vi "Log.vi"(8 "error in (no error)":errorcluster, 10 "MB session in":refnum<class "MB_Master.lvclass">, 11 "DAM0404D in":refnum<class "DAM0404D.lvclass">) -> (0 "error out":errorcluster, 3 "DAM0404D out":refnum<class "DAM0404D.lvclass">)   [LabVIEW 2016, in "DAM0404D.lvlib" / "DAM0404D.lvclass"]
uses:
  DAM0404D.lvclass
  <vilib>/Plasmionique/MB Master/MB_Master/MB_Master.lvclass
  DAM0404D.lvclass/DAM0404D.ctl
  <vilib>/Plasmionique/MB Master/MB_ADU/MB_ADU.lvclass/MB_ADU.ctl
  <vilib>/Plasmionique/MB Master/MB_ADU/Read TX Timestamp.vi
  <vilib>/Plasmionique/MB Master/MB_ADU/Read TX Data.vi
  <vilib>/Plasmionique/MB Master/MB_ADU/Read RX Timestamp.vi
  <vilib>/Plasmionique/MB Master/MB_ADU/Read RX Data.vi
  <vilib>/Plasmionique/MB Master/MB_ADU/MB_ADU.lvclass
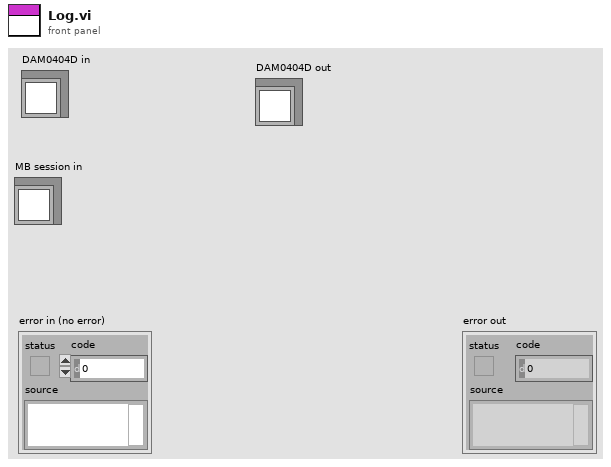
[diagram p1: front panel]
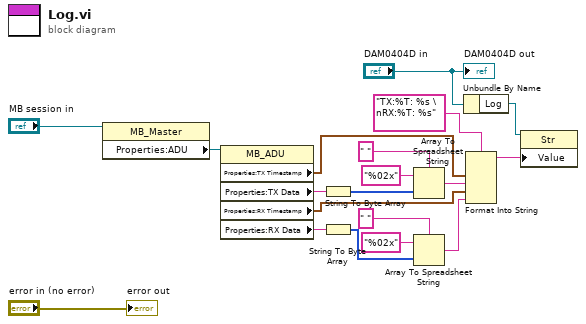
[diagram p0: block diagram]
diagram:
  n1 = property class="MB_Master"(reference="MB session in") -> ("Properties:ADU"=w18:refnum<class "MB_ADU.lvclass">)  [unwired: 1 in, 2 out]
  n2 = property class="MB_ADU"(reference=w18) -> ("Properties:TX Timestamp"=w17:timestamp, "Properties:TX Data"=w2:string, "Properties:RX Timestamp"=w16:timestamp, "Properties:RX Data"=w10:string)  [unwired: 1 in, 2 out]
  n3 = String To Byte Array(string=w2) -> (unsigned byte array=w3:u8[])
  n4 = String To Byte Array(string=w10) -> (unsigned byte array=w9:u8[])
  n5 = Array To Spreadsheet String(delimiter (Tab)=" ", array=w3, 3:"%02x" ("format string")) -> (spreadsheet string=w1:string)
  n6 = Array To Spreadsheet String(delimiter (Tab)=" ", array=w9, 3:"%02x" ("format string")) -> (spreadsheet string=w6:string)
  n7 = Unbundle By Name("DAM0404D in") -> ("Log"=w15:refnum<vi>)
  n8 = Format Into String(format string="TX:%T: %s \nRX:%T: %s", w17, w1, w16, w6) -> (resulting string=w14:string)  [unwired: 2 in, 1 out]
  n9 = property class="Str"(reference=w15, "Value"=w14) -> ()  [unwired: 1 in, 2 out]
  "DAM0404D out" <- "DAM0404D in"
  "error out" <- "error in (no error)"
